vi "Copy_Error_Files.vi"(8 "error in (no error)":errorcluster, 10 "preview only?":bool, 11 "AB_Application in":refnum<class "AB_Application.lvclass">) -> (0 "error out":errorcluster, 2 "copied error files":path[](array[path]), 3 "AB_Application out":refnum<class "AB_Application.lvclass">)   [LabVIEW 2020, in "AB_Application.lvclass"]
uses:
  <vilib>/AppBuilder/AB_Classes/Application/AB_Application.lvclass
  e:/builds/penguin/labview/branches/2020/dev/dist/vi.lib/AppBuilder/AB_Classes/TargetFile/AB_Targetfile.lvclass
  <vilib>/AppBuilder/AB_Classes/Application/AB_Application.lvclass/AB_Application.ctl
  <vilib>/AppBuilder/AB_Classes/TargetFile/AB_Targetfile.lvclass
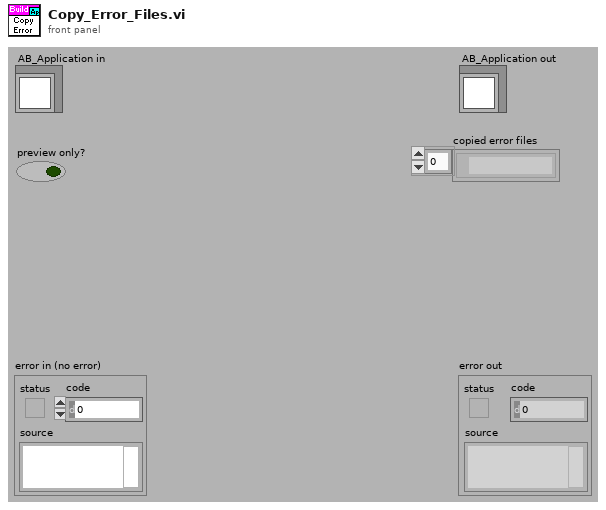
[diagram p1: front panel]
types:
  T1 = enum32{"invalid OS target", "Mac OS", "Windows 3.1", "Windows 95/NT", "Solaris 1", "Solaris 2", "HP-UX", "PowerMAX", "Linux", "Irix", "Rhapsody", "BeOS", "AIX", "OSF1", "VxWorks", "PharLap", "Carbon", "RTX", "Windows x64", "Linux x64", "Mac OS X x64"}
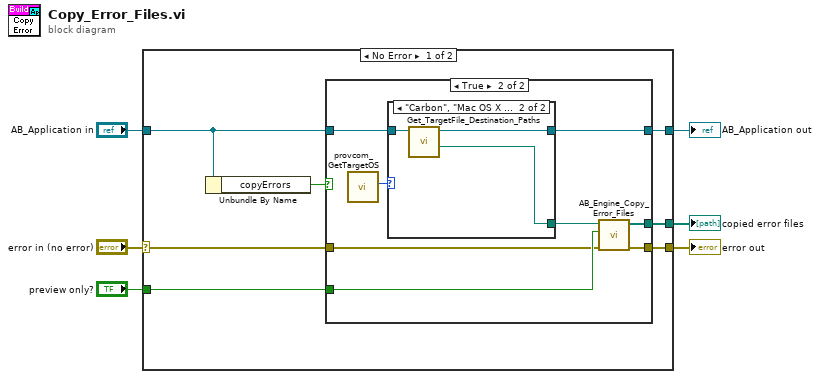
[diagram p0: block diagram]
diagram:
  n1 = case shown="No Error" "error in (no error)" {
    selector: "error in (no error)" -> [w12 w29]
    tunnel: [w11 w29] -> w5
    tunnel: [w7 w28] -> w3
    tunnel: "AB_Application in" -> [w8 w28]
    tunnel: "preview only?" -> [w10 _]
    tunnel: [w9 _] -> w1
    frame No Error {
      n2 = Unbundle By Name(w8) -> ("copyErrors"=w13:bool)
      n3 = case shown="True" w13 {
        tunnel: w12 -> [w15 w20]
        tunnel: [w15 w23] -> w11
        tunnel: w10 -> [_ w22]
        tunnel: [_ w21] -> w9
        tunnel: w8 -> [w14 w18]
        tunnel: [w14 w17] -> w7
        frame False {
        }
        frame True {
          n4 = call <resource>:"provcom_GetTargetOS.vi"() -> ("App.TargetOS"=w19:T1)  [unwired: 11 out]
          n5 = case shown="\"Carbon\", \"Mac OS X x64\"" w19 {
            tunnel: w18 -> [w24 w27]
            tunnel: [w24 w26] -> w17
            tunnel: [_ w25] -> w16
            frame Default {
              # "Empy path causes subVI to locate RTE path. This is what we do on Windows and Linux."
            }
            frame "Carbon", "Mac OS X x64" {
              n6 = call <vilib>:"Get_TargetFile_Destination_Paths.vi"("AB_Targetfile in"=w27) -> ("support path"=w25:path, "AB_Targetfile out"=w26:refnum<class "AB_Application.lvclass">)  [unwired: 6 in, 3 out]
            }
          }
          n7 = call <vilib>:"AB_Engine_Copy_Error_Files.vi"("error in (no error)"=w20, "preview only?"=w22, "Error destination path"=w16) -> ("error out"=w23:errorcluster, "copied error files"=w21:path[])  [unwired: 7 in]
        }
      }
    }
    frame Error {
    }
  }
  "error out" <- w5
  "AB_Application out" <- w3
  "copied error files" <- w1
